vi "PCF8563.vi"() -> ()   [LabVIEW 2024]
uses:
  <vilib>/MakerHub/LINX/Public/Utilities/Open Local.vi
  <vilib>/MakerHub/LINX/LMH-LINX.lvlib
panel:
  out "Year":u16
  out "Month":u16
  out "Weekday":string
  out "Day":u16
  out "Hour":u16
  out "Minute":u16
  in  "Set Date & Time":bool
  out "Second":u16
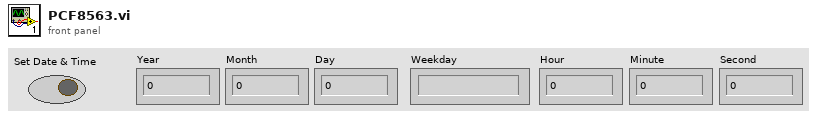
[diagram p1: front panel]
types:
  T1 = cluster{"I2C Slave Address":u8, "I2C Channel":u8}
  T2 = typedef "LMH-LINX.lvlib/LINX Ref.ctl" = cluster{"IO":T3, "Interface":T4, "LINX Device Config":T5}
  T3 = typedef "LMH-LINX.lvlib/Platform.ctl" = enum16{"Remote", "Local"}
  T4 = typedef "LMH-LINX.lvlib/Interface.ctl" = enum16{"Serial", "TCP"}
  T5 = typedef "LMH-LINX.lvlib/Device.lvlib/LINX Device Config.ctl" = cluster{"Interface":T4, "COM Port":refnum<visa-resource-name>, "TCP Configuration":T6, "Device Family":u8, "Device ID":u8, "Device Name":string, "TCP Ref":refnum<k5>, "Channels":T7}
  T6 = typedef "LMH-LINX.lvlib/Device.lvlib/TCP Config.ctl" = cluster{"IP Address":string, "Port":u16}
  T7 = typedef "LMH-LINX.lvlib/Channels.ctl" = cluster{"DI":u8[], "DO":u8[], "AI":u8[], "AO":u8[], "PWM":u8[], "QE":u8[], "UART":u8[], "I2C 2":u8[], "SPI":u8[], "CAN":u8[], "Servo":u8[], "AI Ref (V)":dbl, "AI Resolution (Bits)":u8, "AO Ref (V)":dbl, "AO Resolution (Bits)":u8}
  T8 = typedef "LVDateTimeRec.ctl" = cluster{"fractional second":dbl, "second":i32, "minute":i32, "hour":i32, "day of month":i32, "month":i32, "year":i32, "day of week":i32, "day of year":i32, "DST":i32}
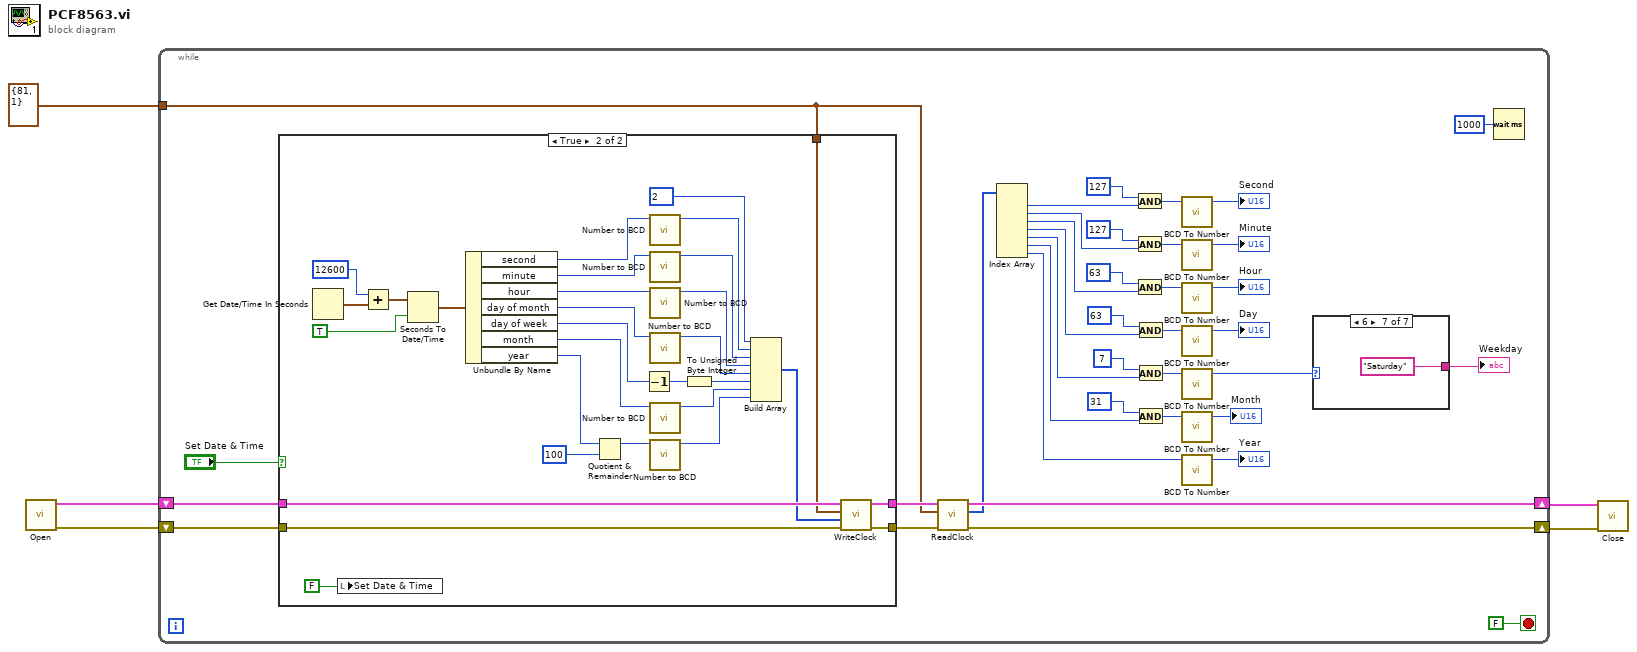
[diagram p0: block diagram]
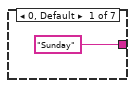
[diagram p2: hidden frame]
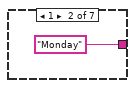
[diagram p3: hidden frame]
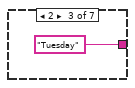
[diagram p4: hidden frame]
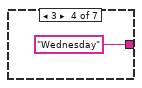
[diagram p5: hidden frame]
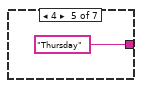
[diagram p6: hidden frame]
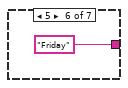
[diagram p7: hidden frame]
diagram:
  n1 = call-poly <vilib>:"Open.vi"() -> ("Error Out"=w4:errorcluster, "LINX Resource"=w5:T2)  [unwired: 9 in, 1 out]
  n2 = while {
    tunnel: T1 {"I2C Slave Address"=81, "I2C Channel"=1} ("Cluster") -> [w32]
    shift-right: [w37] -> w3
    shift-left: w5 -> [w42]
    shift-right: [w36] -> w2
    shift-left: w4 -> [w41]
    stop <- FALSE stop-if-true
    n3 = case shown="True" "Set Date & Time" {
      tunnel: w42 -> [w52 w82]
      tunnel: w41 -> [w51 w81]
      tunnel: w32 -> [_ w80]
      tunnel: [w52 w79] -> w39
      tunnel: [w51 w78] -> w38
      frame False {
      }
      frame True {
        n4 = Get Date/Time In Seconds() -> (seconds since 1Jan1904=w76:timestamp)
        n5 = local write "Set Date & Time"(FALSE ("Set Date & Time")) -> ()
        n6 = Add(x=12600, y=w76) -> (x+y=w54:timestamp)
        n7 = Seconds To Date/Time(time stamp (now)=w54, to UTC (F)=TRUE) -> (date time rec=w55:T8)
        n8 = Unbundle By Name(w55) -> ("second"=w75:i32, "minute"=w74:i32, "hour"=w73:i32, "day of month"=w72:i32, "day of week"=w65:i32, "month"=w71:i32, "year"=w70:i32)
        n9 = Quotient & Remainder(x=w70, y=100) -> (x-y*floor(x/y)=w59:i32)  [unwired: 1 out]
        n10 = Decrement(x=w65) -> (x-1=w62:i32)
        n11 = call "Number to BCD.vi"("Number"=w75) -> ("BCD"=w69:u8)  [unwired: 10 in]
        n12 = call "Number to BCD.vi"("Number"=w74) -> ("BCD"=w68:u8)  [unwired: 10 in]
        n13 = call "Number to BCD.vi"("Number"=w73) -> ("BCD"=w67:u8)  [unwired: 10 in]
        n14 = call "Number to BCD.vi"("Number"=w72) -> ("BCD"=w66:u8)  [unwired: 10 in]
        n15 = call "Number to BCD.vi"("Number"=w71) -> ("BCD"=w64:u8)  [unwired: 10 in]
        n16 = call "Number to BCD.vi"("Number"=w59) -> ("BCD"=w63:u8)  [unwired: 10 in]
        n17 = To Unsigned Byte Integer(number=w62) -> (unsigned 8bit integer=w60:u8)
        n18 = Build Array(u8 2 ("x"), w69, w68, w67, w66, w60, w64, w63) -> (w57:u8[])
        n19 = call "WriteClock.vi"("Error In"=w81, "Time & Date"=w57, "Cluster"=w80, "LINX Resource"=w82) -> ("Error Out"=w78:errorcluster, "LINX Resource"=w79:T2)  [unwired: 4 in]
      }
    }
    n20 = call "ReadClock.vi"("Error In"=w38, "Cluster"=w32, "LINX Resource"=w39) -> ("Error Out"=w36:errorcluster, "Clock"=w33:u8[], "LINX Resource"=w37:T2)  [unwired: 4 in]
    n21 = Index Array(array=w33) -> (element #1=w34:u8, element #2=w24:u8, element #3=w23:u8, element #4=w16:u8, element #5=w15:u8, element #6=w14:u8, element #7=w13:u8)  [unwired: 7 in]
    n22 = And(x=u8 127, y=w34) -> (x .and. y?=w30:u8)
    n23 = And(x=u8 127, y=w24) -> (x .and. y?=w27:u8)
    n24 = And(x=u8 63, y=w23) -> (x .and. y?=w26:u8)
    n25 = And(x=u8 63, y=w16) -> (x .and. y?=w17:u8)
    n26 = And(x=u8 7, y=w15) -> (x .and. y?=w20:u8)
    n27 = And(x=u8 31, y=w14) -> (x .and. y?=w21:u8)
    n28 = call "BCD To Number.vi"("BCD"=w30) -> ("Number"=→"Second":u16)  [unwired: 8 in]
    n29 = call "BCD To Number.vi"("BCD"=w27) -> ("Number"=→"Minute":u16)  [unwired: 8 in]
    n30 = call "BCD To Number.vi"("BCD"=w26) -> ("Number"=→"Hour":u16)  [unwired: 8 in]
    n31 = call "BCD To Number.vi"("BCD"=w17) -> ("Number"=→"Day":u16)  [unwired: 8 in]
    n32 = call "BCD To Number.vi"("BCD"=w20) -> ("Number"=w7:u16)  [unwired: 8 in]
    n33 = call "BCD To Number.vi"("BCD"=w21) -> ("Number"=→"Month":u16)  [unwired: 8 in]
    n34 = call "BCD To Number.vi"("BCD"=w13) -> ("Number"=→"Year":u16)  [unwired: 8 in]
    n35 = case shown="6" w7 {
      tunnel: ["Sunday" "Monday" "Tuesday" "Wednesday" "Thursday" "Friday" "Saturday"] -> w6
      frame 0, Default {
      }
      frame 1 {
      }
      frame 2 {
      }
      frame 3 {
      }
      frame 4 {
      }
      frame 5 {
      }
      frame 6 {
      }
    }
    "Weekday" <- w6
    n36 = Wait (ms)(milliseconds to wait=u32 1000) -> ()  [unwired: 1 out]
  }
  n37 = call <vilib>:"Close.vi"("Error In"=w2, "LINX Resource"=w3) -> ()  [unwired: 9 in, 1 out]
